vi "Stop.vi"(8 "error in (no error)":errorcluster) -> (0 "error out":errorcluster)   [LabVIEW 2018, in "GLog.lvlib" / "Registry.lvlib"]
uses:
  Registry.lvlib
  Registry Message.ctl
  Registry Actions.ctl
  Registry Actions Event.vi
panel:
  # "Connector Pane"
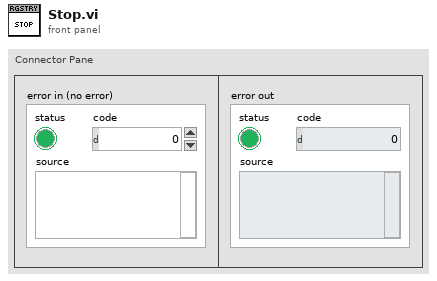
[diagram p1: front panel]
types:
  T1 = typedef "GLog.lvlib/Registry.lvlib/Registry Message.ctl" = cluster{"action":T2, "data":variant, "return notifier":refnum<notifier>}
  T2 = typedef "GLog.lvlib/Registry.lvlib/Registry Actions.ctl" = enum16{"Register", "Log", "Enable", "Enable All", "Disable", "Disable All", "List", "Unregister", "Unregister All", "Shutdown"}
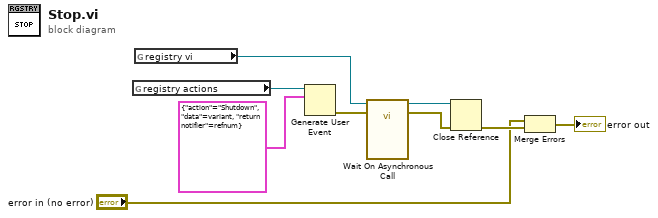
[diagram p0: block diagram]
diagram:
  n1 = global read "Registry Actions Event.vi" "registry actions"() -> (w9:refnum<user-event>)
  n2 = global read "Registry Actions Event.vi" "registry vi"() -> (w7:refnum<vi>)
  n3 = Generate User Event(user event=w9, event data cluster=T1 {"action"=enum."Shutdown", "data"=variant, "return notifier"=refnum} ("event data")) -> (error out=w6:errorcluster)  [unwired: 2 in, 1 out]
  n4 = call-by-ref "Wait On Asynchronous Call"(reference=w7, error in=w6) -> (reference out=w5:refnum<vi>, error out=w4:errorcluster)  [unwired: 12 in]
  n5 = Close Reference(reference=w5, error in (no error)=w4) -> (error out=w3:errorcluster)
  n6 = Merge Errors("error in (no error)", w3) -> (→"error out":errorcluster)
